vi "register websocket handler.vi"(8 "error in":errorcluster, 10 "websocket user plugin":refnum<class "websocket user plugin.lvclass">, 11 "http responder in":refnum<class "http responder.lvclass">) -> (0 "error out":errorcluster, 3 "http responder out":refnum<class "http responder.lvclass">)   [LabVIEW 2016, in "websocket upgrade handler.lvclass"]
uses:
  websocket upgrade handler.lvclass
  user plugin/websocket user plugin.lvclass
  HTTP responder/http responder.lvclass
  HTTP responder/http upgrade callback.ctl
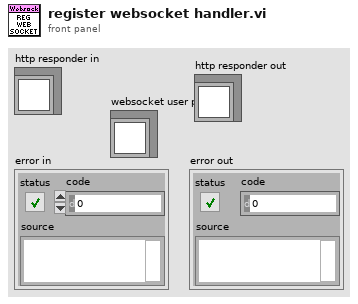
[diagram p1: front panel]
types:
  T1 = typedef "http responder.lvclass/http upgrade callback.ctl" = cluster{"callback":refnum<vi>, "parameters":variant, "unregister callback":refnum<vi>}
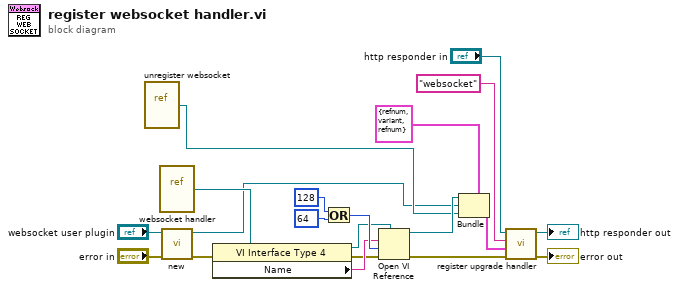
[diagram p0: block diagram]
diagram:
  n1 = vi-ref "unregister websocket.vi"() -> (w3:refnum<vi>)
  n2 = vi-ref "websocket handler.vi"() -> (w6:refnum<vi>)
  n3 = call "new.vi"("error in"="error in", "websocket user plugin"="websocket user plugin") -> ("error out"=w11:errorcluster, "websocket upgrade handler out"=w1:refnum<class "websocket upgrade handler.lvclass">)  [unwired: 8 in]
  n4 = property class="VI Interface Type 4"(reference=w6, error in=w11) -> (reference out=w16:refnum<vi>, error out=w14:errorcluster, "Name"=w15:string)
  n5 = Or(x=128 ("options"), y=64 ("options")) -> (x .or. y?=w17:i32)
  n6 = Open VI Reference(type specifier VI Refnum (for type only)=w16, vi path=w15, options=w17, error in (no error)=w14) -> (vi reference=w4:refnum<vi>, error out=w20:errorcluster)  [unwired: 2 in]
  n7 = Bundle(cluster=T1 {"callback"=refnum, "parameters"=variant, "unregister callback"=refnum} ("callback"), "callback"=w4, "parameters"=w1, "unregister callback"=w3) -> (w2:T1)
  n8 = call "register upgrade handler.vi"("error in"=w20, "callback"=w2, "protocol"="websocket" ("name"), "http responder in"="http responder in") -> ("error out"=→"error out":errorcluster, "http responder out"=→"http responder out":refnum<class "http responder.lvclass">)  [unwired: 6 in]
